vi "Remove Error Cluster Attribute.vi"(10 "attribute name":string, 11 "error in":errorcluster) -> (2 "deleted?":bool, 3 "error out":errorcluster)   [LabVIEW 2020, in "Multi Error Cluster.lvlib"]
doc: "Removes an attribute from an error cluster."
uses:
  <vilib>/MultiError/TokenizeJSON/Multi Error Cluster.lvlib
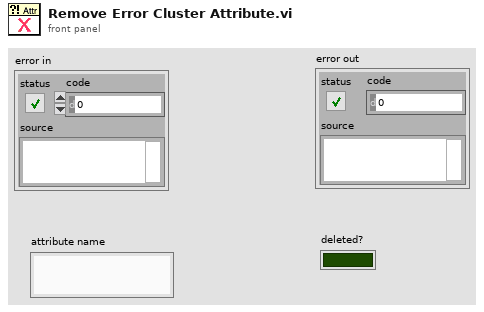
[diagram p1: front panel]
types:
  T1 = typedef "Multi Error Cluster.lvlib/JSON Token Values.ctl" = enum32{"array begin", "array end", "object begin", "object end", "value", "invalid", "name"}
  T2 = typedef "Multi Error Cluster.lvlib/JSON Token Descriptor.ctl" = cluster{"match string":string, "raw token type":T3, "byte offset ":i32}
  T3 = typedef "Multi Error Cluster.lvlib/JSON Raw Token Values.ctl" = enum32{"{", "}", "[", "]", ",", ":", "\"", "number", "string", "true", "false", "null", "invalid"}
  T4 = typedef "Multi Error Cluster.lvlib/JSON Object Descriptor.ctl" = cluster{"begin info":T2, "end info":T2, "begin Index":i32, "end Index":i32}
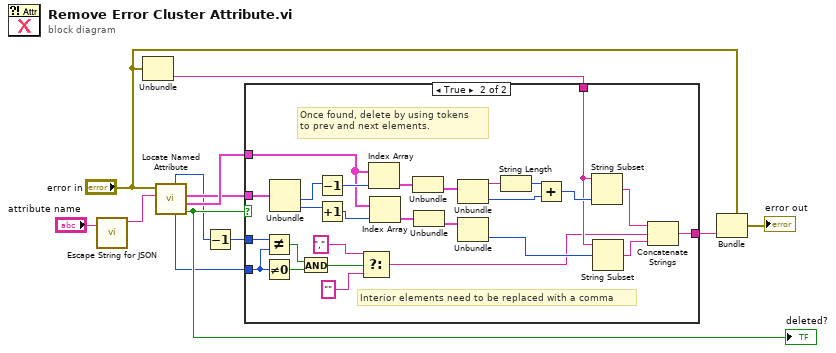
[diagram p0: block diagram]
diagram:
  n1 = call <vilib>:"Escape String for JSON.vi"("string"="attribute name") -> ("quoted string"=w1:string)  [unwired: 10 in]
  n2 = Unbundle("error in") -> ("source"=w11:string)  [unwired: 2 out]
  n3 = call <vilib>:"Locate Named Attribute.vi"("attribute name"=w1, "error"="error in") -> ("found"=w6:bool, "attribute tokens"=w8:cluster{"token type":T1, T2}[], "JSON Object Descriptor"=w7:T4, "attr index"=w5:i32, "attributes"=w4:i32)  [unwired: 5 in]
  "deleted?" <- w6
  n4 = Decrement(x=w4) -> (x-1=w3:i32)
  n5 = case shown="True" w6 {
    tunnel: w11 -> [w13 w25]
    tunnel: [w13 w22] -> w10
    tunnel: w7 -> [_ w40]
    tunnel: w5 -> [_ w21]
    tunnel: w3 -> [_ w39]
    tunnel: w8 -> [_ w35]
    frame False {
    }
    frame True {
      # "Interior elements need to be replaced with a comma"
      # "Once found, delete by using tokens\nto prev and next elements."
      n6 = Not Equal?(x=w39, y=w21) -> (x != y?=w19:bool)
      n7 = Not Equal To 0?(x=w21) -> (x != 0?=w20:bool)
      n8 = Unbundle(w40) -> ("begin Index"=w38:i32, "end Index"=w37:i32)  [unwired: 2 out]
      n9 = And(x=w19, y=w20) -> (x .and. y?=w16:bool)
      n10 = Decrement(x=w38) -> (x-1=w36:i32)
      n11 = Increment(x=w37) -> (x+1=w34:i32)
      n12 = Select(t=",", s=w16, f="") -> (s? t:f=w14:string)
      n13 = Index Array(array=w35, index=w36) -> (element=w33:cluster{"token type":T1, T2})
      n14 = Index Array(array=w35, index=w34) -> (element=w32:cluster{"token type":T1, T2})
      n15 = Unbundle(w33) -> (w31:T2)  [unwired: 1 out]
      n16 = Unbundle(w32) -> (w30:T2)  [unwired: 1 out]
      n17 = Unbundle(w31) -> ("match string"=w29:string, "byte offset"=w27:i32)  [unwired: 1 out]
      n18 = Unbundle(w30) -> ("byte offset"=w24:i32)  [unwired: 2 out]
      n19 = String Length(string=w29) -> (length=w28:i32)
      n20 = Add(x=w28, y=w27) -> (x+y=w26:i32)
      n21 = String Subset(string=w25, length (rest)=w26) -> (substring=w23:string)  [unwired: 1 in]
      n22 = String Subset(string=w25, offset (0)=w24) -> (substring=w15:string)  [unwired: 1 in]
      n23 = Concatenate Strings(w23, w14, w15) -> (w22:string)
    }
  }
  n24 = Bundle(cluster="error in", "source"=w10) -> (→"error out":errorcluster)  [unwired: 2 in]
